vi "export_image.vi"(8 "error in (no error)":errorcluster, 9 "Refnum in":T1, 10 "path in":path, 11 "map size in":cluster{dbl, dbl, dbl, dbl}) -> (0 "error out":errorcluster, 1 "Refnum out":T1, 2 "path out":path, 3 "map size out":cluster{dbl, dbl, dbl, dbl})   [LabVIEW 2012]
uses:
  <vilib>/vision/Image Controls.llb/IMAQ Image.ctl
panel:
  in  "Add bar":bool
  in  "Save":bool
  in  "Exit":bool
  out "Image":T1(plugin-control)
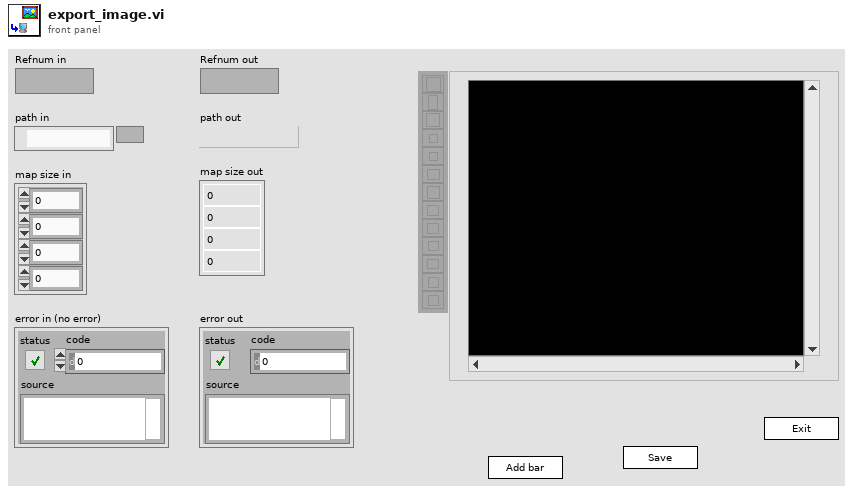
[diagram p1: front panel]
types:
  T1 = typedef "IMAQ Image.ctl" = refnum<image>
  T2 = typedef "Image Type" = u32
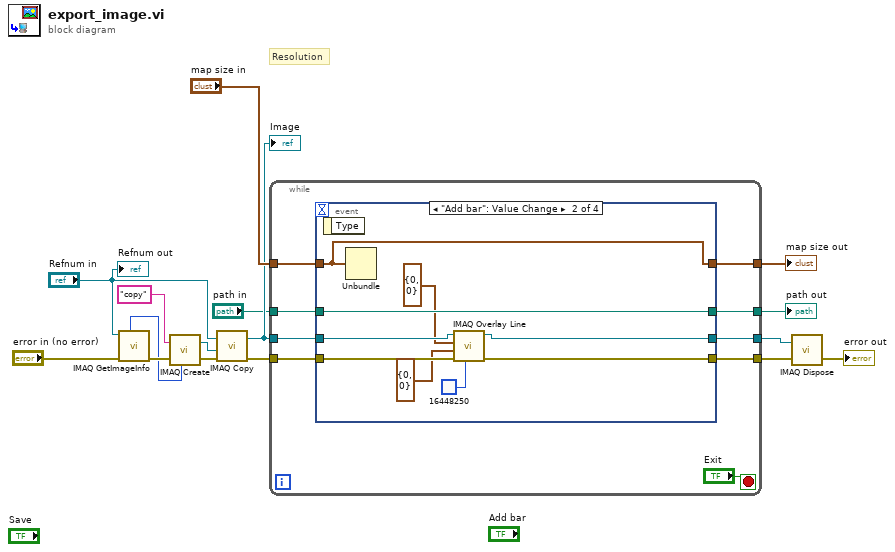
[diagram p0: block diagram]
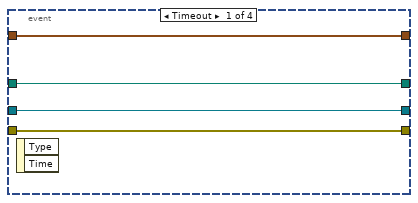
[diagram p2: hidden frame]
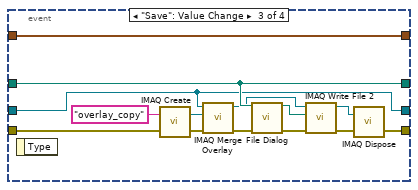
[diagram p3: hidden frame]
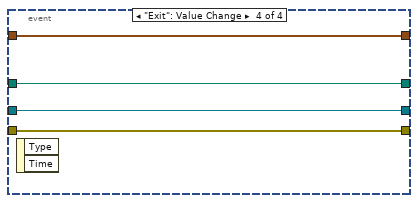
[diagram p4: hidden frame]
diagram:
  # "Resolution"
  n1 = call "IMAQ GetImageInfo"("error in (no error)"="error in (no error)", "Image"="Refnum in") -> ("error out"=w14:errorcluster, "Image Type"=w11:T2)  [unwired: 2 in, 6 out]
  n2 = call "IMAQ Create"("Image Name"="copy", "Image Type"=w11, "error in (no error)"=w14) -> ("New Image"=w12:T1, "error out"=w8:errorcluster)  [unwired: 2 in]
  n3 = call "IMAQ Copy"("error in (no error)"=w8, "Image Dst"=w12, "Image Src"="Refnum in") -> ("error out"=w7:errorcluster, "Image Dst Out"=w6:T1)  [unwired: 3 in]
  "Image" <- w6
  n4 = while {
    tunnel: w7 -> [w22]
    tunnel: [w23] -> w4
    tunnel: "map size in" -> [w24]
    tunnel: [w21] -> w16
    tunnel: w6 -> [w20]
    tunnel: [w19] -> w5
    tunnel: "path in" -> [w18]
    tunnel: [w17] -> w1
    stop <- "Exit" stop-if-true
    n5 = event shown="[1] \"Add bar\": Value Change" {
      selector: _ -> [_ _ _ _]
      dyn-events: _ -> [_ _ _ _]
      timeout: _ -> [_ _ _ _]
      tunnel: w24 -> [w28 w33 w50 w56]
      tunnel: [w29 w37 w39 w54] -> w23
      tunnel: w22 -> [w29 w38 w48 w54]
      tunnel: [w28 w33 w50 w56] -> w21
      tunnel: w20 -> [w27 w36 w42 w55]
      tunnel: [w27 w35 w42 w55] -> w19
      tunnel: w18 -> [w26 w34 w49 w53]
      tunnel: [w26 w34 w49 w53] -> w17
      event Timeout {
        n6 = event-data() -> ()  [unwired: 1 in, 2 out]
      }
      event "Add bar": Value Change {
        n7 = event-data() -> ()  [unwired: 1 in, 1 out]
        n8 = Unbundle(w33) -> ()  [unwired: 4 out]
        n9 = call "IMAQ Overlay Line"("Color"=u32 16448250, "error in (no error)"=w38, "End Point"=cluster{"X":i32, "Y":i32} {"X"=0, "Y"=0}, "Start Point"=cluster{"X":i32, "Y":i32} {"X"=0, "Y"=0}, "Image"=w36) -> ("error out"=w37:errorcluster, "Image Out"=w35:T1)  [unwired: 5 in]
      }
      event "Save": Value Change {
        n10 = event-data() -> ()  [unwired: 1 in, 1 out]
        n11 = call "IMAQ Create"("Image Name"="overlay_copy", "error in (no error)"=w48) -> ("New Image"=w46:T1, "error out"=w44:errorcluster)  [unwired: 3 in]
        n12 = call "IMAQ Merge Overlay"("error in (no error)"=w44, "Image Dst"=w46, "Image Src"=w42) -> ("error out"=w43:errorcluster, "Image Dst Out"=w45:T1)  [unwired: 7 in]
        n13 = call "File Dialog"("start path"=w49, "error in"=w43) -> ("selected path"=w51:path, "error out"=w52:errorcluster)  [unwired: 10 in, 2 out]
        n14 = call-poly "IMAQ Write File 2"("error in (no error)"=w52, "File Path"=w51, "Image"=w45) -> ("error out"=w40:errorcluster, "Image Out (duplicate)"=w41:T1)  [unwired: 7 in]
        n15 = call "IMAQ Dispose"("Image"=w41, "error in (no error)"=w40) -> ("error out"=w39:errorcluster)  [unwired: 4 in]
      }
      event "Exit": Value Change {
        n16 = event-data() -> ()  [unwired: 1 in, 2 out]
      }
    }
  }
  "map size out" <- w16
  "path out" <- w1
  n17 = call "IMAQ Dispose"("Image"=w5, "error in (no error)"=w4) -> ("error out"=→"error out":errorcluster)  [unwired: 4 in]
  "Refnum out" <- "Refnum in"
